vi "Sine.Generate.Convert.vi"(11 "Settings":T2={"Amplitude"=0.0, "Offset"=0.0, "Frequency"=5000.0}) -> (3 "Settings":T1={"Amplitude"=0.0, "Offset"=0.0, "Periods/Tick"=0.0002500000409781933})   [LabVIEW 2015, in "Speciality FPGA IO.lvlib"]
uses:
  Speciality FPGA IO.lvlib
  Types/Sine.Generate.Convert.Settings.ctl
  Types/Sine.Generate.Settings.ctl
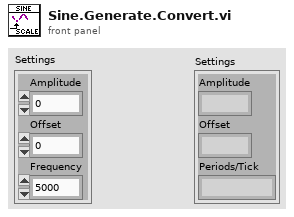
[diagram p1: front panel]
types:
  T1 = typedef "Speciality FPGA IO.lvlib/Sine.Generate.Settings.ctl" = cluster{"Amplitude":fxp<+/-,32,8>, "Offset":fxp<+/-,32,8>, "Periods/Tick":fxp<+,32,0>}
  T2 = typedef "Speciality FPGA IO.lvlib/Sine.Generate.Convert.Settings.ctl" = cluster{"Amplitude":sgl, "Offset":sgl, "Frequency":sgl}
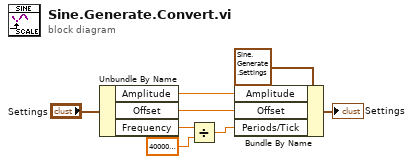
[diagram p0: block diagram]
diagram:
  n1 = Unbundle By Name("Settings") -> ("Amplitude"=w4:sgl, "Offset"=w3:sgl, "Frequency"=w2:sgl)
  n2 = Divide(x=w2, y=sgl 40000000.0) -> (x/y=w6:sgl)
  n3 = Bundle By Name(cluster=T1 {"Amplitude"=0.0, "Offset"=0.0, "Periods/Tick"=0.0002500000409781933} ("Settings"), "Amplitude"=w4, "Offset"=w3, "Periods/Tick"=w6) -> (→"Settings":T1)
